vi "Set Caption - Add To Library Checkbox.vi"(8 "error in":errorcluster, 9 "Owner Filename (including extension)":string, 10 "User VI Owner Status":T1, 11 "Add To Owner":refnum<vi>) -> (0 "error out":errorcluster)   [LabVIEW 2022 SP3]
doc: "Configures the check box:\n1. Enables or Disables and greyes out the checkbox\n2. Sets the caption"
uses:
  Owner Status (enum).ctl
panel:
  # "Development\ncontrols/indicators useful for development and testing, but which are not outputs of the VI"
  # "Input\nInputs to the VI"
  # "Output\nOutputs of the VI"
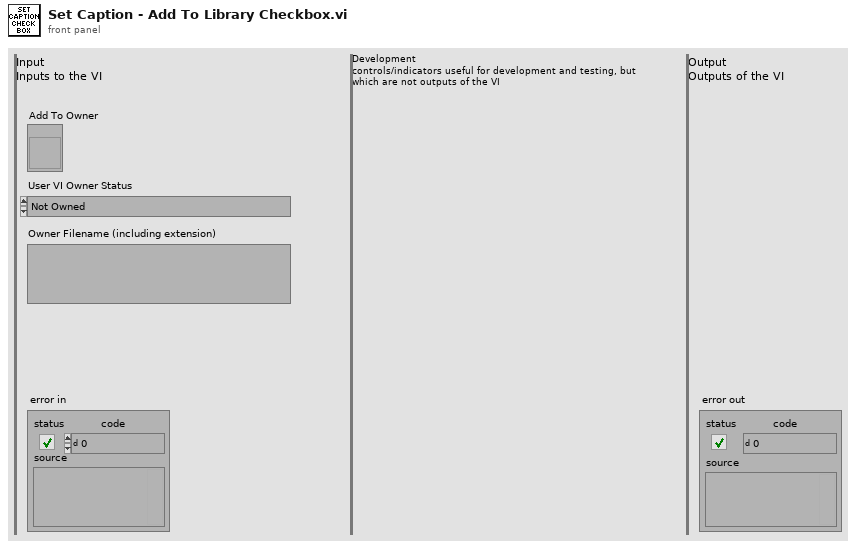
[diagram p1: front panel]
types:
  T1 = typedef "Owner Status (enum).ctl" = enum16{"Not Owned", "Owned by Library (lvlib)", "Owned by Class (lvclass)"}
  T2 = enum8{"Enabled", "Disabled", "Disabled and Grayed Out"}
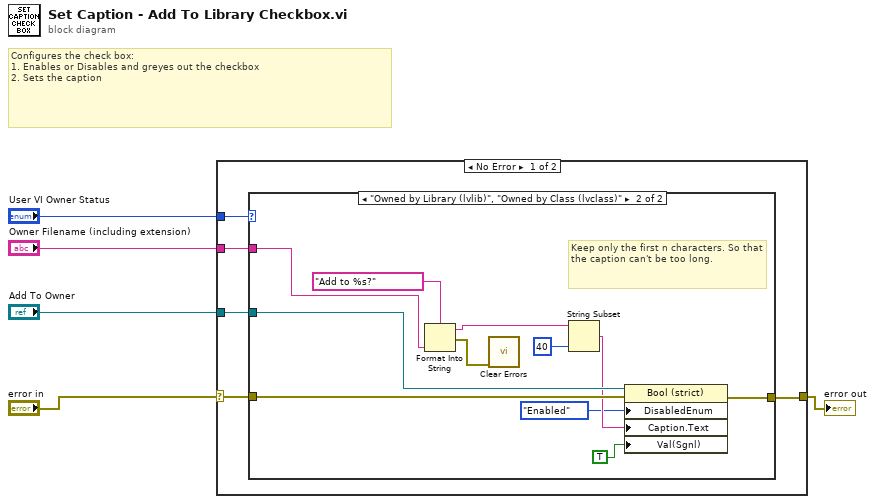
[diagram p0: block diagram]
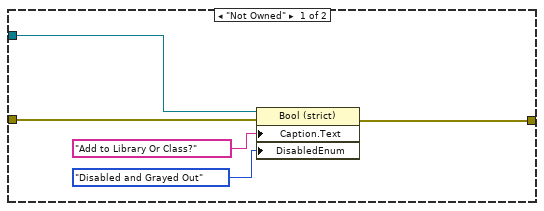
[diagram p2: hidden frame]
diagram:
  # "Configures the check box:\n1. Enables or Disables and greyes out the checkbox\n2. Sets the caption"
  n1 = case shown="No Error" "error in" {
    selector: "error in" -> [w9 w27]
    tunnel: [w7 w27] -> w4
    tunnel: "Add To Owner" -> [w8 _]
    tunnel: "User VI Owner Status" -> [w10 _]
    tunnel: "Owner Filename (including extension)" -> [w6 _]
    frame No Error {
      n2 = case shown="\"Owned by Library (lvlib)\", \"Owned by Class (lvclass)\"" w10 {
        tunnel: w9 -> [w15 w26]
        tunnel: w8 -> [w14 w25]
        tunnel: [w12 w24] -> w7
        tunnel: w6 -> [_ w22]
        frame "Not Owned" {
          n3 = property class="Bool (strict)"(reference=w14, error in=w15, "Caption.Text"="Add to Library Or Class?", "DisabledEnum"=T2."Disabled and Grayed Out" ("Disabled")) -> (error out=w12:errorcluster)  [unwired: 1 out]
        }
        frame "Owned by Library (lvlib)", "Owned by Class (lvclass)" {
          # "Keep only the first n characters. So that the caption can't be too long."
          n4 = Format Into String(format string="Add to %s?" ("Caption.Text"), w22) -> (resulting string=w20:string, error out=w21:errorcluster)  [unwired: 2 in]
          n5 = call <vilib>:"Clear Errors.vi"("error in (no error)"=w21) -> ()  [unwired: 5 in, 2 out]
          n6 = String Subset(string=w20, length (rest)=40 ("length (rest)")) -> (substring=w17:string)  [unwired: 1 in]
          n7 = property class="Bool (strict)"(reference=w25, error in=w26, "DisabledEnum"=T2."Enabled" ("Disabled"), "Caption.Text"=w17, "Val(Sgnl)"=TRUE ("Value")) -> (error out=w24:errorcluster)  [unwired: 1 out]
        }
      }
    }
    frame Error {
    }
  }
  "error out" <- w4
